vi "Get Tag.vi"(6 "Namespace":string, 8 "error in (no error)":errorcluster, 10 "Name":string) -> (0 "error out":errorcluster, 1 "found":bool, 2 "Tag Ref out":refnum<data-value>)   [LabVIEW 2020, in "Tag Engine.lvlib"]
doc: "Lookup the reference of a Tag.\n\nOptionally specify a namespace, which is prepended to the tag name (colon separator).\n\nIf the tag is not found, the found output is false and Error 5602 is returned."
uses:
  Tag Engine.lvlib
  Core/Tag Core.lvclass
  Tag/Tag.lvclass
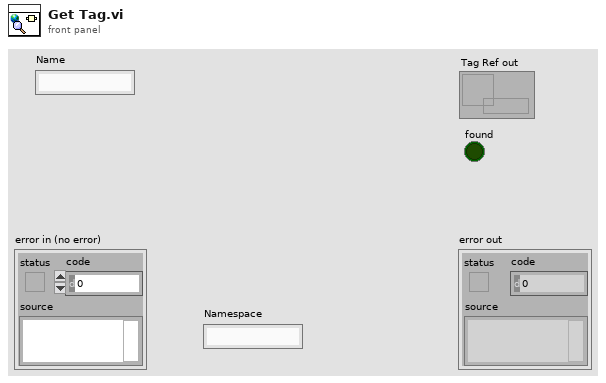
[diagram p1: front panel]
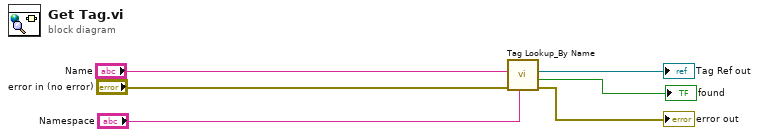
[diagram p0: block diagram]
diagram:
  n1 = call "Tag Lookup_By Name.vi"("Namespace"="Namespace", "error in (no error)"="error in (no error)", "Name"="Name") -> ("error out"=→"error out":errorcluster, "found"=→"found":bool, "Tag Ref out"=→"Tag Ref out":refnum<data-value>)  [unwired: 6 in]
